vi "findSC-DATA-IR-SD.vi"(2 "II channel":u16[][](array[numeric]), 3 "I channel":u16[][](array[numeric])) -> (0 "II channel":u16[][](array[numeric]), 1 "I channel":u16[][](array[numeric]))   [LabVIEW 2015]
uses:
  globalVarSD.vi
panel:
  out "Numérique":i32
  out "out":dbl[](graph) caption="Data Values"
  out "in":dbl[](graph) caption="Data Values"
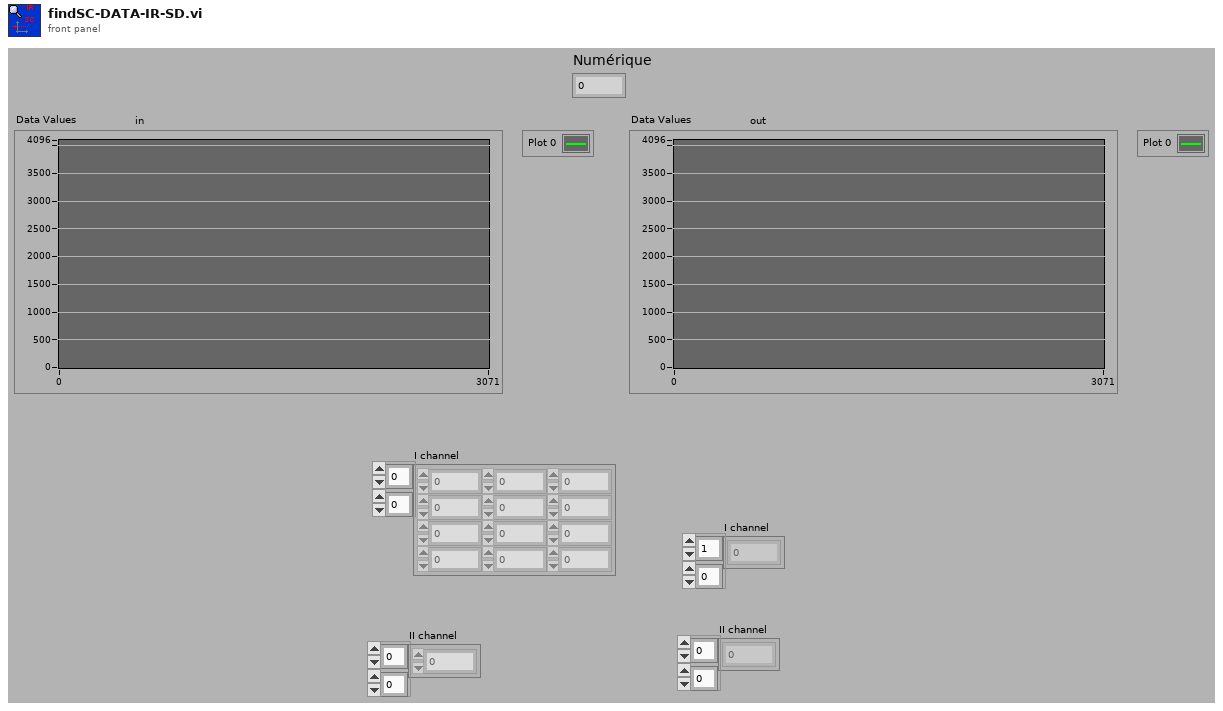
[diagram p1: front panel]
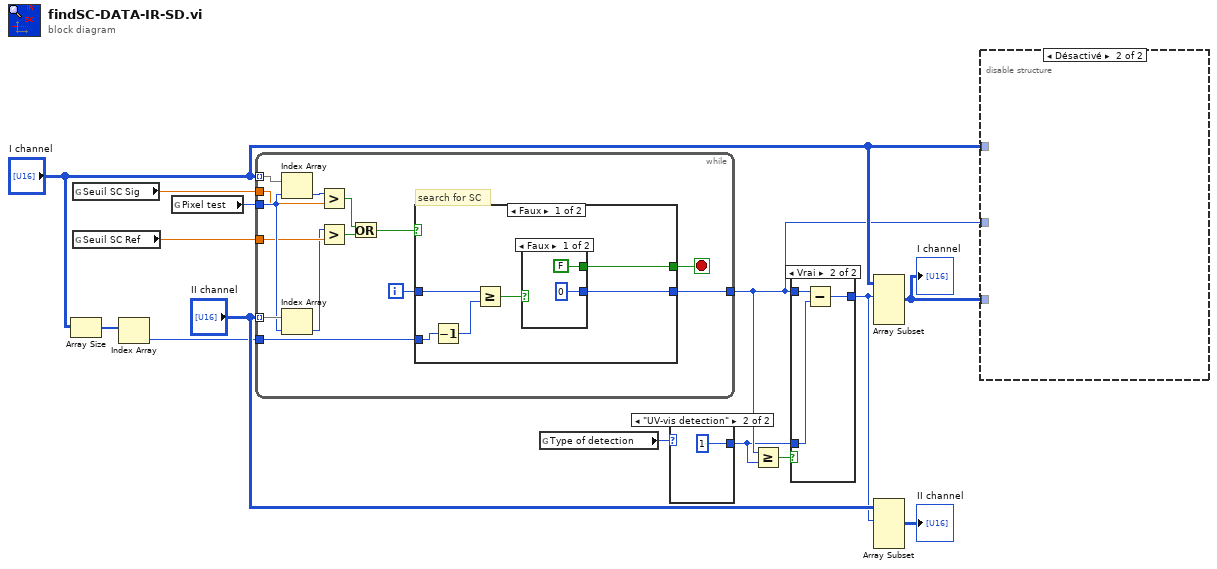
[diagram p0: block diagram]
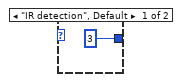
[diagram p2: hidden frame]
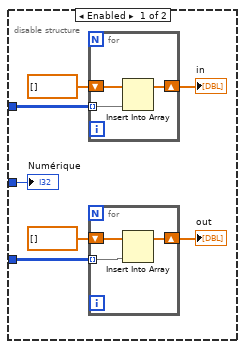
[diagram p4: hidden frame]
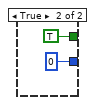
[diagram p5: hidden frame]
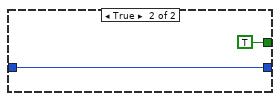
[diagram p6: hidden frame]
diagram:
  n1 = Array Size(array="I channel") -> (size(s)=w6:i32[])
  n2 = global read "globalVarSD.vi" "Seuil SC Sig"() -> (w14:dbl)
  n3 = global read "globalVarSD.vi" "Seuil SC Ref"() -> (w13:dbl)
  n4 = Index Array(array=w6) -> (element=w5:i32)  [unwired: 1 in]
  n5 = global read "globalVarSD.vi" "Pixel test"() -> (w12:u32)
  n6 = while {
    tunnel: "I channel" -> [w26] mode=indexing
    tunnel: "II channel" -> [w25] mode=indexing
    tunnel: w14 -> [w23]
    tunnel: w13 -> [w21]
    tunnel: w12 -> [w24]
    tunnel: [w17] -> w4
    tunnel: w5 -> [w15]
    i -> [w16]
    stop <- w19 stop-if-true
    # "search for SC"
    n7 = Index Array(array=w26, index=w24) -> (element=w22:u16)
    n8 = Index Array(array=w25, index=w24) -> (element=w20:u16)
    n9 = Greater?(x=w22, y=w23) -> (0:w28:bool)
    n10 = Greater?(x=w20, y=w21) -> (0:w27:bool)
    n11 = Or(x=w28, y=w27) -> (x .or. y?=w18:bool)
    n12 = case shown="Faux" w18 {
      tunnel: [w29 TRUE] -> w19
      tunnel: [w30 w39] -> w17
      tunnel: w16 -> [w34 w39]
      tunnel: w15 -> [w33 _]
      frame False {
        n13 = Decrement(x=w33) -> (x-1=w32:i32)
        n14 = Greater Or Equal?(x=w34, y=w32) -> (x >= y?=w31:bool)
        n15 = case shown="Faux" w31 {
          tunnel: [0 0] -> w30
          tunnel: [FALSE TRUE] -> w29
          frame False {
          }
          frame True {
          }
        }
      }
      frame True {
      }
    }
  }
  n16 = global read "globalVarSD.vi" "Type of detection"() -> (w2:enum32{"IR detection", "UV-vis detection"})
  n17 = case shown="\"UV-vis detection\"" w2 {
    tunnel: [3 ("y") 1 ("y")] -> w1
    frame "IR detection", Default {
    }
    frame "UV-vis detection" {
    }
  }
  n18 = Greater Or Equal?(x=w4, y=w1) -> (x >= y?=w9:bool)
  n19 = case shown="Vrai" w9 {
    tunnel: [w43 w45] -> w8
    tunnel: w4 -> [w43 w46]
    tunnel: w1 -> [_ w44]
    frame False {
    }
    frame True {
      n20 = Subtract(x=w46, y=w44) -> (x-y=w45:i32)
    }
  }
  n21 = Array Subset(array="I channel", index (row)=w8) -> (w3:u16[][])  [unwired: 3 in]
  "I channel" <- w3
  n22 = Array Subset(array="II channel", index (row)=w8) -> (→"II channel":u16[][])  [unwired: 3 in]
  n23 = disable-structure shown="Désactivé" {
    disable-tunnel: "I channel" -> [w51 _]
    disable-tunnel: w3 -> [w48 _]
    disable-tunnel: w4 -> [w47 _]
    frame Enabled {
      n24 = for {
        tunnel: w51 -> [w57] mode=indexing
        shift-right: [w58] -> w52
        shift-left: dbl[] [] ("tableau") -> [w59]
        n25 = Insert Into Array(array=w59, new element=w57) -> (w58:dbl[])  [unwired: 1 in]
      }
      "in" <- w52
      n26 = for {
        tunnel: w48 -> [w54] mode=indexing
        shift-right: [w55] -> w50
        shift-left: dbl[] [] ("tableau") -> [w56]
        n27 = Insert Into Array(array=w56, new element=w54) -> (w55:dbl[])  [unwired: 1 in]
      }
      "out" <- w50
      "Numérique" <- w47
    }
    frame Disabled {
    }
  }
